vi "Populate.vi"(8 "error in (no error)":errorcluster, 9 "Values":string[](array[string]), 10 "Names":string[](array[string]), 11 "Action Interface in":refnum<class>) -> (0 "error out":errorcluster, 1 "Success?":bool, 3 "Action Interface out":refnum<class>)   [LabVIEW 2019, in "ProjectBuilder.lvlib" / "Project Action.lvclass"]
doc: "Populate private data from string arrays if the given class uses the interface."
uses:
  Class/Project Action/Project Action.lvclass
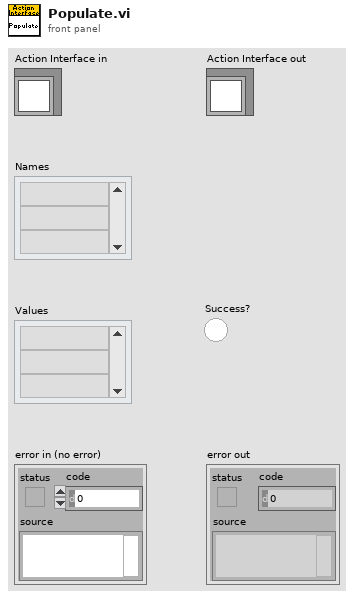
[diagram p1: front panel]
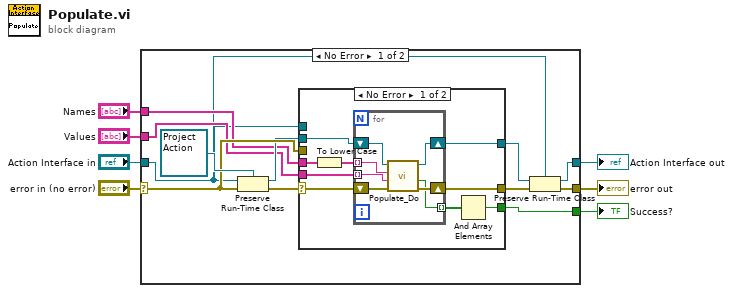
[diagram p0: block diagram]
diagram:
  n1 = case shown="No Error" "error in (no error)" {
    selector: "error in (no error)" -> [w17 w39]
    tunnel: [w9 w39] -> w6
    tunnel: [w11 w38] -> w4
    tunnel: "Action Interface in" -> [w8 w38]
    tunnel: "Names" -> [w15 _]
    tunnel: "Values" -> [w14 _]
    tunnel: [w13 _] -> w1
    frame No Error {
      n2 = Preserve Run-Time Class(object in=w8, error in=w17, 2:refnum<class "Project Action.lvclass"> refnum ("ProjectBuilder.lvlib:Project Action Interface.lvclass")) -> (object out=w16:refnum<class "Project Action.lvclass">, error out=w18:errorcluster)
      n3 = case shown="No Error" w18 {
        selector: w18 -> [w23 _]
        tunnel: [w24 w37] -> w12
        tunnel: w8 -> [_ w37]
        tunnel: [w22 w36] -> w10
        tunnel: w17 -> [_ w36]
        tunnel: w16 -> [w28 _]
        tunnel: w15 -> [w27 _]
        tunnel: w14 -> [w26 _]
        tunnel: [w20 _] -> w13
        frame No Error {
          n4 = To Lower Case(string=w27) -> (all lower case string=w25:string[])
          n5 = for {
            tunnel: w26 -> [w34] mode=indexing
            tunnel: w25 -> [w33] mode=indexing
            shift-right: [w32] -> w24
            shift-left: w28 -> [w35]
            shift-right: [w30] -> w22
            shift-left: w23 -> [w31]
            tunnel: [w29] -> w21 mode=indexing
            n6 = call-dynamic "Populate_Do.vi"("error in (no error)"=w31, "Value"=w34, "Lower case name"=w33, "Action in"=w35) -> ("error out"=w30:errorcluster, "Success?"=w29:bool, "Action out"=w32:refnum<class "Project Action.lvclass">)  [unwired: 5 in]
          }
          n7 = And Array Elements(Boolean array=w21) -> (logical AND=w20:bool)
        }
        frame Error {
        }
      }
      n8 = Preserve Run-Time Class(object in=w12, error in=w10, 2:w8) -> (object out=w11:refnum<class>, error out=w9:errorcluster)
    }
    frame Error {
    }
  }
  "error out" <- w6
  "Action Interface out" <- w4
  "Success?" <- w1
